vi "Items Count.vi"(8 "error in (no error)":errorcluster caption="错误输入（无错误）", 11 "HashTable 输入":refnum<class "HashTable.lvclass"> caption="DNL_LabVIEW Object in") -> (0 "error out":errorcluster caption="错误输出", 2 "Count":i32, 3 "HashTable 输出":refnum<class "HashTable.lvclass"> caption="DNL_LabVIEW Object out")   [LabVIEW 2012, in "HashTable.lvclass"]
uses:
  HashTable.lvclass
  HashTable.lvclass/HashTable.ctl
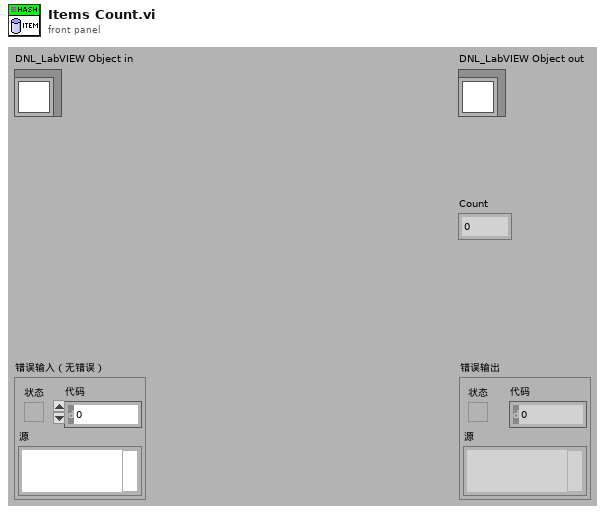
[diagram p1: front panel]
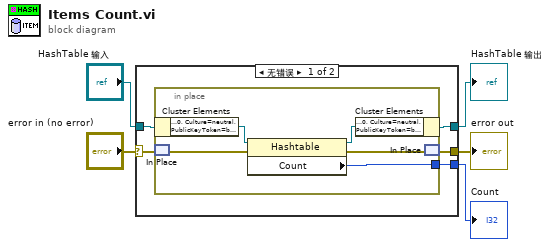
[diagram p0: block diagram]
diagram:
  n1 = case shown="无错误" "error in (no error)" {
    selector: "error in (no error)" -> [w8 w17]
    tunnel: [w7 w17] -> w4
    tunnel: [w9 w16] -> w2
    tunnel: "HashTable 输入" -> [w10 w16]
    tunnel: [w6 _] -> w1
    frame No Error {
      n2 = in-place {
        in-place-border: [w13] -> w6
        n3 = in-place-cluster #1(w10) -> ("HashTable"=w15:refnum<k24>)
        n4 = in-place-match #2(w8) -> (w14:errorcluster)
        n5 = property class="Hashtable"(reference=w15, error in=w14) -> (reference out=w11:refnum<k24>, error out=w12:errorcluster, "Count"=w13:i32)
        n6 = in-place-cluster #1("HashTable"=w11) -> (w9:refnum<class "HashTable.lvclass">)
        n7 = in-place-match #2(w12) -> (w7:errorcluster)
      }
    }
    frame Error {
    }
  }
  "error out" <- w4
  "HashTable 输出" <- w2
  "Count" <- w1
